vi "Main.vi"() -> ()   [LabVIEW 2020]
uses:
  Actor 1 - State machine/Actor 1 - State machine/Actor 1 - State machine.lvclass
  C:/Program Files/National Instruments/LabVIEW 2020/vi.lib/ActorFramework/Actor/Actor.lvclass
  <vilib>/ActorFramework/Actor/Actor.lvclass
panel:
  out "error out":errorcluster
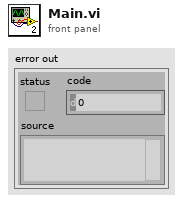
[diagram p1: front panel]
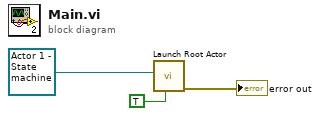
[diagram p0: block diagram]
diagram:
  n1 = call <vilib>:"Launch Root Actor.vi"("Open Actor Core front panel? (F)"=TRUE, "Actor"=refnum<class "Actor 1 - State machine.lvclass"> refnum ("Actor 1 - State machine.lvlib:Actor 1 - State machine.lvclass")) -> ("error out"=→"error out":errorcluster)  [unwired: 8 in, 1 out]
